vi "SEND STATUS.vi"(7 "ELEMENT":T1, 8 "error in (no error)":errorcluster) -> (0 "error out":errorcluster)   [LabVIEW 2019]
uses:
  TypeDef/DEVICE NAME.ctl
  APLUS Driver/TypeDef/cluster STATUS UPDATE.ctl
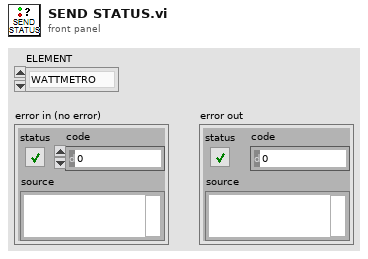
[diagram p1: front panel]
types:
  T1 = typedef "DEVICE NAME.ctl" = enum16{"WATTMETRO", "APLUS", "PLC BANCO 1", "PLC RACK", "PLC BANCO 2", "PS", "NI cDAQ", "RESISTOMAT"}
  T2 = cluster{"Array of elements":cluster{"String":string, "variant":variant}[], "Single element":cluster{"String":string, "variant":variant}, "enque at\nopposite end (F)":bool, "no replications (F)":bool}
  T3 = typedef "cluster STATUS UPDATE.ctl" = cluster{"ELEMENT":enum16{"WATTMETRO", "APLUS", "PLC BANCO 1", "PLC RACK", "PLC BANCO 2", "PS", "NI cDAQ", "RESISTOMAT"}, "ERROR?":bool}
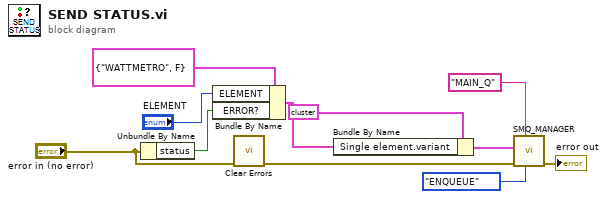
[diagram p0: block diagram]
diagram:
  n1 = Unbundle By Name("error in (no error)") -> ("status"=w8:bool)
  n2 = Bundle By Name(cluster=T3 {"ELEMENT"=enum."WATTMETRO", "ERROR?"=FALSE}, "ELEMENT"="ELEMENT", "ERROR?"=w8) -> (w9:T3)
  n3 = call <vilib>:"Clear Errors.vi"("error in (no error)"="error in (no error)") -> ("error out"=w2:errorcluster)  [unwired: 5 in, 1 out]
  n4 = Bundle By Name(cluster=T2 {"Array of elements"=[], "Single element"={"String"="STATUS UPDATE", "variant"=variant}, "enque at\nopposite end (F)"=FALSE, "no replications (F)"=FALSE} ("Enqueue cluster"), "Single element.variant"=w9) -> (w10:T2)
  n5 = call <userlib>:"SMQ_MANAGER.vi"("Function"=enum16{"INITIALIZE", "ENQUEUE", "STOP ALL"}."ENQUEUE", "Queue name"="MAIN_Q", "error in (no error)"=w2, "Enqueue cluster"=w10) -> ("error out"=→"error out":errorcluster)  [unwired: 7 in]
